vi "Reset.vi"(8 "error in (no error)":errorcluster, 11 "DataLogger in":refnum<class "DataLogger.lvclass">) -> (0 "error out":errorcluster, 3 "DataLogger out":refnum<class "DataLogger.lvclass">)   [LabVIEW 2020, in "VolatusDataLogger.lvlib" / "DataLogger.lvclass"]
uses:
  DataLogger.lvclass
  DataLogger.lvclass/DataLogger.ctl
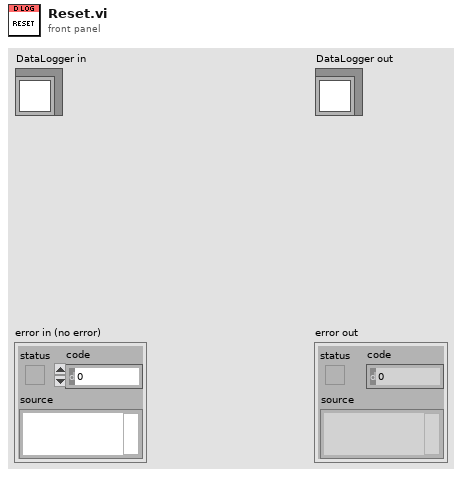
[diagram p1: front panel]
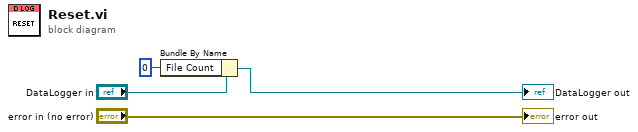
[diagram p0: block diagram]
diagram:
  n1 = Bundle By Name(cluster="DataLogger in", "File Count"=0) -> (→"DataLogger out":refnum<class "DataLogger.lvclass">)
  "error out" <- "error in (no error)"
